vi "Set SV.vi"(8 "error in (no error)":errorcluster, 9 "SV Value":variant, 10 "SV Name":string, 11 "SV_Publisher in":refnum<class "SV_Publisher.lvclass">) -> (0 "error out":errorcluster, 3 "SV_Publisher out":refnum<class "SV_Publisher.lvclass">)   [LabVIEW 2019, in "SV_Publisher.lvclass"]
uses:
  SV_Publisher.lvclass
  Data.ctl
  SV_Publisher.lvclass/SV_Publisher.ctl
  1ae5d02c-efd0-450a-8aa4-8388e25d05bc.vi
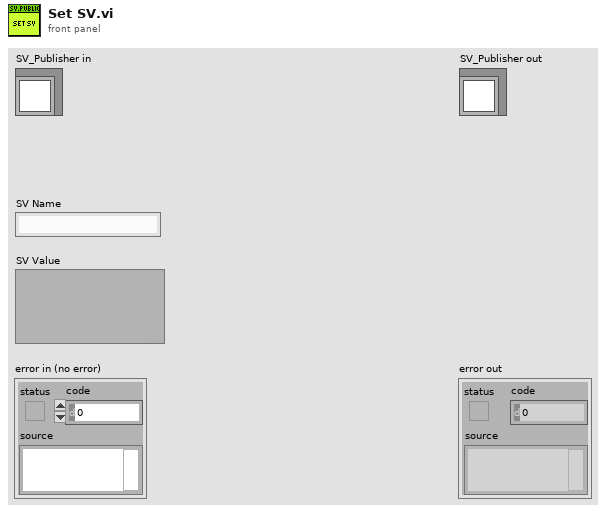
[diagram p1: front panel]
types:
  T1 = typedef "SV_Publisher.lvclass/Data.ctl" = cluster{"Name":string, "Value":variant}
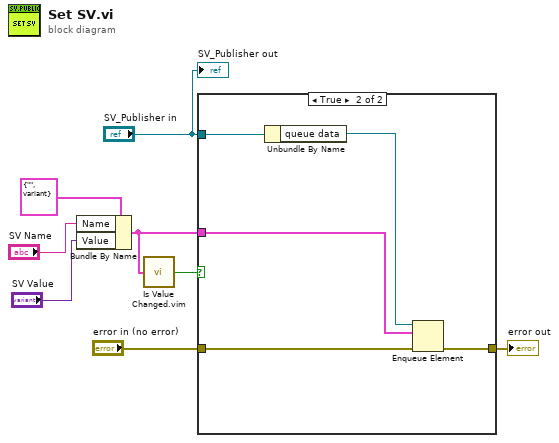
[diagram p0: block diagram]
diagram:
  n1 = Bundle By Name(cluster=T1 {"Name"="", "Value"=variant} ("element"), "Name"="SV Name", "Value"="SV Value") -> (w1:T1)
  n2 = call "Is Value Changed.vim"("value"=w1) -> ("changed or first call?"=w2:bool)
  n3 = case shown="True" w2 {
    tunnel: "SV_Publisher in" -> [_ w14]
    tunnel: "error in (no error)" -> [w9 w12]
    tunnel: [w9 w11] -> w6
    tunnel: w1 -> [_ w10]
    frame False {
    }
    frame True {
      n4 = Unbundle By Name(w14) -> ("queue data"=w13:refnum<queue>)
      n5 = Enqueue Element(queue=w13, element=w10, error in (no error)=w12) -> (error out=w11:errorcluster)  [unwired: 1 in, 2 out]
    }
  }
  "error out" <- w6
  "SV_Publisher out" <- "SV_Publisher in"
